vi "seriellFIFORT.vi"() -> ()   [LabVIEW 2010]
uses:
  gvbooleschRT.vi
panel:
  in  "FPGA VI Reference In":refnum<k20>
  in  "AnzahlHorst":i32[](array[numeric])
  out "HorstMW":dbl[](array[numeric])
  in  "HorstSPVorwort":string[](array[string])
  in  "HorstAbfragen":string[](array[string])
  in  "HorstSP":dbl[](array[numeric])
  in  "HorstSP0":dbl[](array[numeric])
  in  "SkalierungsfaktorHorst":dbl[](array[numeric])
  in  "VorwortHorst":string[](array[string])
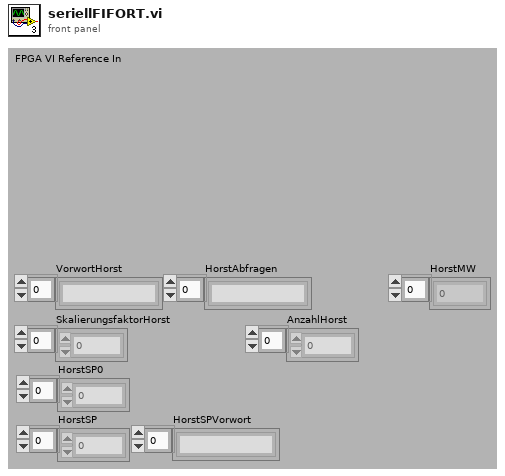
[diagram p1: front panel]
types:
  T1 = cluster{string[], string[], string[], dbl[], dbl[], dbl[]}
  T2 = cluster{"Befehle1":string[], "Befehle2":string[], "Befehle3":string[]}
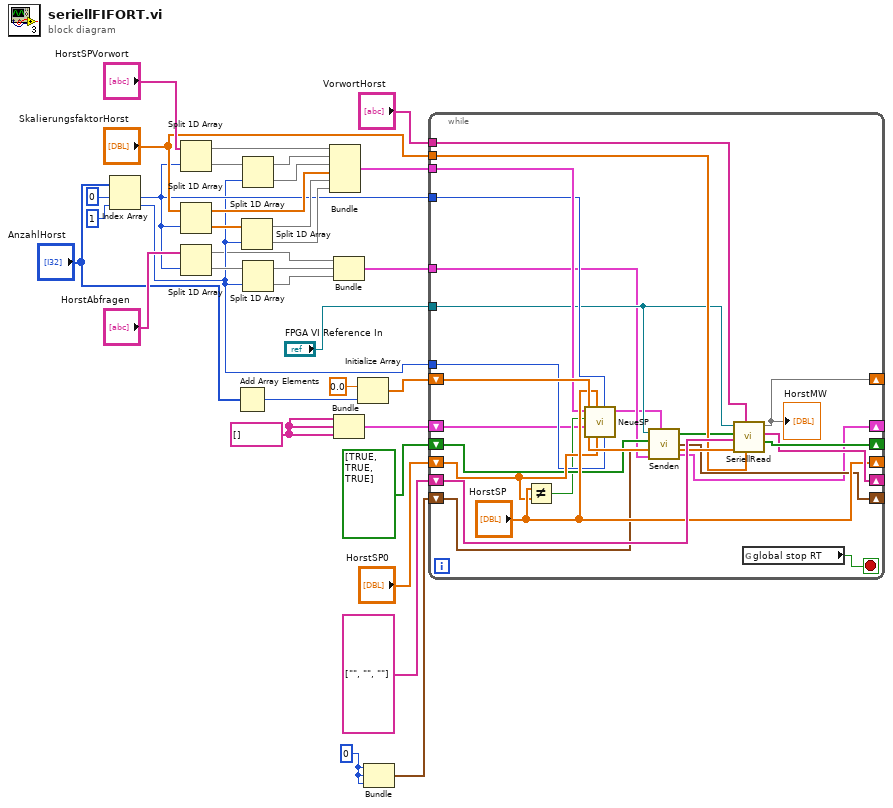
[diagram p0: block diagram]
diagram:
  w9 = 0
  w7 = string[] []
  n1 = Index Array(array="AnzahlHorst", index #1=0 ("Index"), index #2=1 ("Index")) -> (element #1=w16:i32, element #2=w14:i32)
  n2 = Split 1D Array(array="HorstSPVorwort", index=w16) -> (first subarray=w24:string[], second subarray=w27:string[])
  n3 = Split 1D Array(array="SkalierungsfaktorHorst", index=w16) -> (first subarray=w21:dbl[], second subarray=w25:dbl[])
  n4 = Split 1D Array(array="HorstAbfragen", index=w16) -> (first subarray=w13:string[], second subarray=w15:string[])
  n5 = Add Array Elements(numeric array="AnzahlHorst") -> (sum=w4:i32)
  n6 = Split 1D Array(array=w25, index=w14) -> (first subarray=w20:dbl[], second subarray=w19:dbl[])
  n7 = Split 1D Array(array=w27, index=w14) -> (first subarray=w23:string[], second subarray=w22:string[])
  n8 = Split 1D Array(array=w15, index=w14) -> (first subarray=w12:string[], second subarray=w11:string[])
  n9 = Bundle(w24, w23, w22, w21, w20, w19) -> (w18:T1)  [unwired: 1 in]
  n10 = Bundle(w13, w12, w11) -> (w10:cluster{string[], string[], string[]})  [unwired: 1 in]
  n11 = Bundle(w7, w7, w7) -> (w6:cluster{string[], string[], string[]})  [unwired: 1 in]
  n12 = Initialize Array(0.0 ("Element"), w4) -> (w2:dbl[])
  n13 = Bundle(w9, w9, w9) -> (w8:cluster{i32, i32, i32})  [unwired: 1 in]
  n14 = while {
    shift-right: [w57] -> _
    shift-left: bool[] [TRUE, TRUE, TRUE] -> [w43]
    shift-right: ["HorstSP"] -> _
    shift-left: "HorstSP0" -> [w48]
    tunnel: "FPGA VI Reference In" -> [w44]
    shift-right: [w55] -> _
    shift-left: string[] ["", "", ""] -> [w56]
    shift-right: [w54] -> _
    shift-left: w2 -> [w53]
    tunnel: "VorwortHorst" -> [w52]
    tunnel: "SkalierungsfaktorHorst" -> [w51]
    shift-right: [w36] -> _
    shift-left: w6 -> [w38]
    tunnel: w16 -> [w46]
    tunnel: w14 -> [w47]
    tunnel: w18 -> [w49]
    tunnel: w10 -> [w41]
    shift-right: [w40] -> _
    shift-left: w8 -> [w42]
    stop <- w35 stop-if-true
    n15 = Not Equal?(x="HorstSP", y=w48) -> (x != y?=w39:bool)
    n16 = call "NeueSP.vi"("Anzahl2"=w47, "Anzahl1"=w46, "AlteSP"=w48, 7:"NeueSP"="HorstSP", "BefehleCluster"=w38, 10:"NeueSP"=w39, "ClusterFest"=w49) -> ("BefehleCluster"=w37:T2)  [unwired: 4 in]
    n17 = call "Senden.vi"("FPGA VI Reference In"=w44, "BefehlsCluster"=w37, "Senden?"=w43, "Abfragenr.Cluster"=w42, "AbfragenCluster"=w41) -> ("Senden?"=w45:bool[], "Abfragenr.Cluster"=w40:cluster{i32, i32, i32}, "BefehlsCluster"=w36:T2)  [unwired: 1 in]
    n18 = call "SeriellRead.vi"("SkalierungsfaktorHorst"=w51, "VorwortHorst"=w52, 8:w53, "Zwischenspeicher"=w56, "Senden?"=w45, "FPGA VI Reference In"=w44) -> ("Senden?"=w57:bool[], "Zwischenspeicher"=w55:string[], 3:w54)  [unwired: 3 in]
    "HorstMW" <- w54
    n19 = global read "gvbooleschRT.vi" "global stop RT"() -> (w35:bool)
  }
